vi "Init.vi"(9 "Register":refnum<event-registration>, 10 "Addresses Strategy":refnum<class "Addresses Strategy.lvclass">) -> (3 "Base jettl out":refnum<class "Base jettl.lvclass">)   [LabVIEW 2021, in "jettl.lvlib" / "Base jettl.lvclass"]
uses:
  Base jettl.lvclass
  Addresses Strategy/Addresses Strategy/Addresses Strategy.lvclass
  Msg Strategy/Msg Strategy.lvclass
  Base jettl.lvclass/Base jettl.ctl
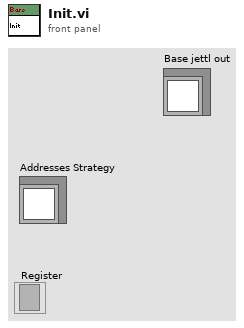
[diagram p1: front panel]
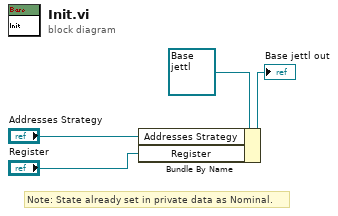
[diagram p0: block diagram]
diagram:
  # "Note: State already set in private data as Nominal."
  n1 = Bundle By Name(cluster=refnum<class "Base jettl.lvclass"> refnum ("jettl Event Actor out"), "Addresses Strategy"="Addresses Strategy", "Register"="Register") -> (→"Base jettl out":refnum<class "Base jettl.lvclass">)
